vi "SVI_NewE2E_VoltageToDAC_IntegerString.vi"(1 "Voltage Limits":cluster{"Maximum":dbl, "Minimum":dbl}, 2 "Divisions (Precision)":i32=4096, 3 "Set Voltage":dbl) -> (0 "DAC Int String":string)   [LabVIEW 2014]
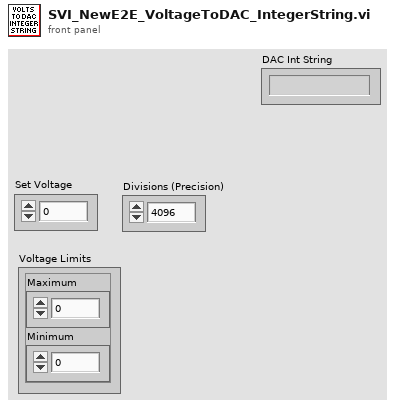
[diagram p1: front panel]
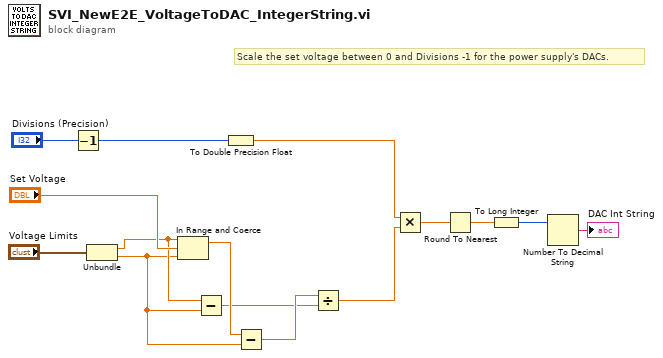
[diagram p0: block diagram]
diagram:
  # "Scale the set voltage between 0 and Divisions -1 for the power supply's DACs."
  n1 = Decrement(x="Divisions (Precision)") -> (x-1=w8:i32)
  n2 = Unbundle("Voltage Limits") -> ("Maximum"=w3:dbl, "Minimum"=w2:dbl)
  n3 = In Range and Coerce(upper limit=w3, x="Set Voltage", lower limit=w2) -> (coerced(x)=w13:dbl)  [unwired: 1 out]
  n4 = Subtract(x=w3, y=w2) -> (x-y=w11:dbl)
  n5 = To Double Precision Float(number=w8) -> (double precision float=w1:dbl)
  n6 = Subtract(x=w13, y=w2) -> (x-y=w12:dbl)
  n7 = Divide(x=w12, y=w11) -> (x/y=w9:dbl)
  n8 = Multiply(x=w1, y=w9) -> (x*y=w7:dbl)
  n9 = Round To Nearest(number=w7) -> (nearest integer value=w6:dbl)
  n10 = To Long Integer(number=w6) -> (32bit integer=w5:i32)
  n11 = Number To Decimal String(number=w5) -> (decimal integer string=→"DAC Int String":string)  [unwired: 1 in]
